vi "Filter Indicator Terms.vi"(11 "Terms[]":refnum<vi>[](array[refnum])) -> (3 "Terms[] out":refnum<vi>[](array[refnum]))   [LabVIEW 2020, in "CSM-Helper.lvclass"]
uses:
  CSM-Helper.lvclass
  de5b2ffe-4539-45f8-a445-c590f0d3ba24.vi
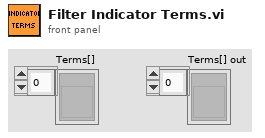
[diagram p1: front panel]
types:
  T1 = typedef "LVPositionTypeDef.ctl" = cluster{"Left":i32, "Top":i32}
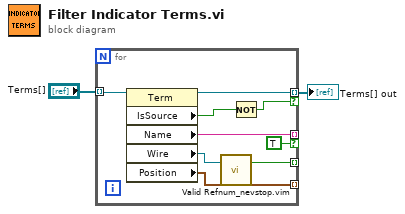
[diagram p0: block diagram]
diagram:
  n1 = for {
    tunnel: "Terms[]" -> [w11] mode=indexing
    tunnel: [w10] -> _ mode=indexing if=TRUE
    tunnel: [w7] -> _ mode=indexing
    tunnel: [w5] -> _ mode=indexing
    tunnel: [w4] -> w1 mode=indexing if=w3
    n2 = property class="Term"(reference=w11) -> (reference out=w4:refnum<vi>, "IsSource"=w9:bool, "Name"=w10:string, "Wire"=w8:refnum<vi>, "Position"=w5:T1)  [unwired: 1 in, 1 out]
    n3 = call "Valid Refnum_nevstop.vim"("number/path/refnum"=w8) -> ("Valid Number/Path/Refnum"=w7:bool)  [unwired: 2 in]
    n4 = Not(x=w9) -> (.not. x?=w3:bool)
  }
  "Terms[] out" <- w1
